vi "enumAttr.vi"() -> ()   [LabVIEW 2016]
uses:
  <vilib>/userdefined/High Color/IMAQdx.ctl
  <vilib>/vision/driver/IMAQdx.llb/IMAQdx Attribute Type.ctl
  <vilib>/vision/driver/NI_Vision_Acquisition_Software.lvlib
panel:
  in  "stop":bool
  out "error out":errorcluster
  out "Attribute Information Array":T2(array[cluster])
  in  "Session In":T3
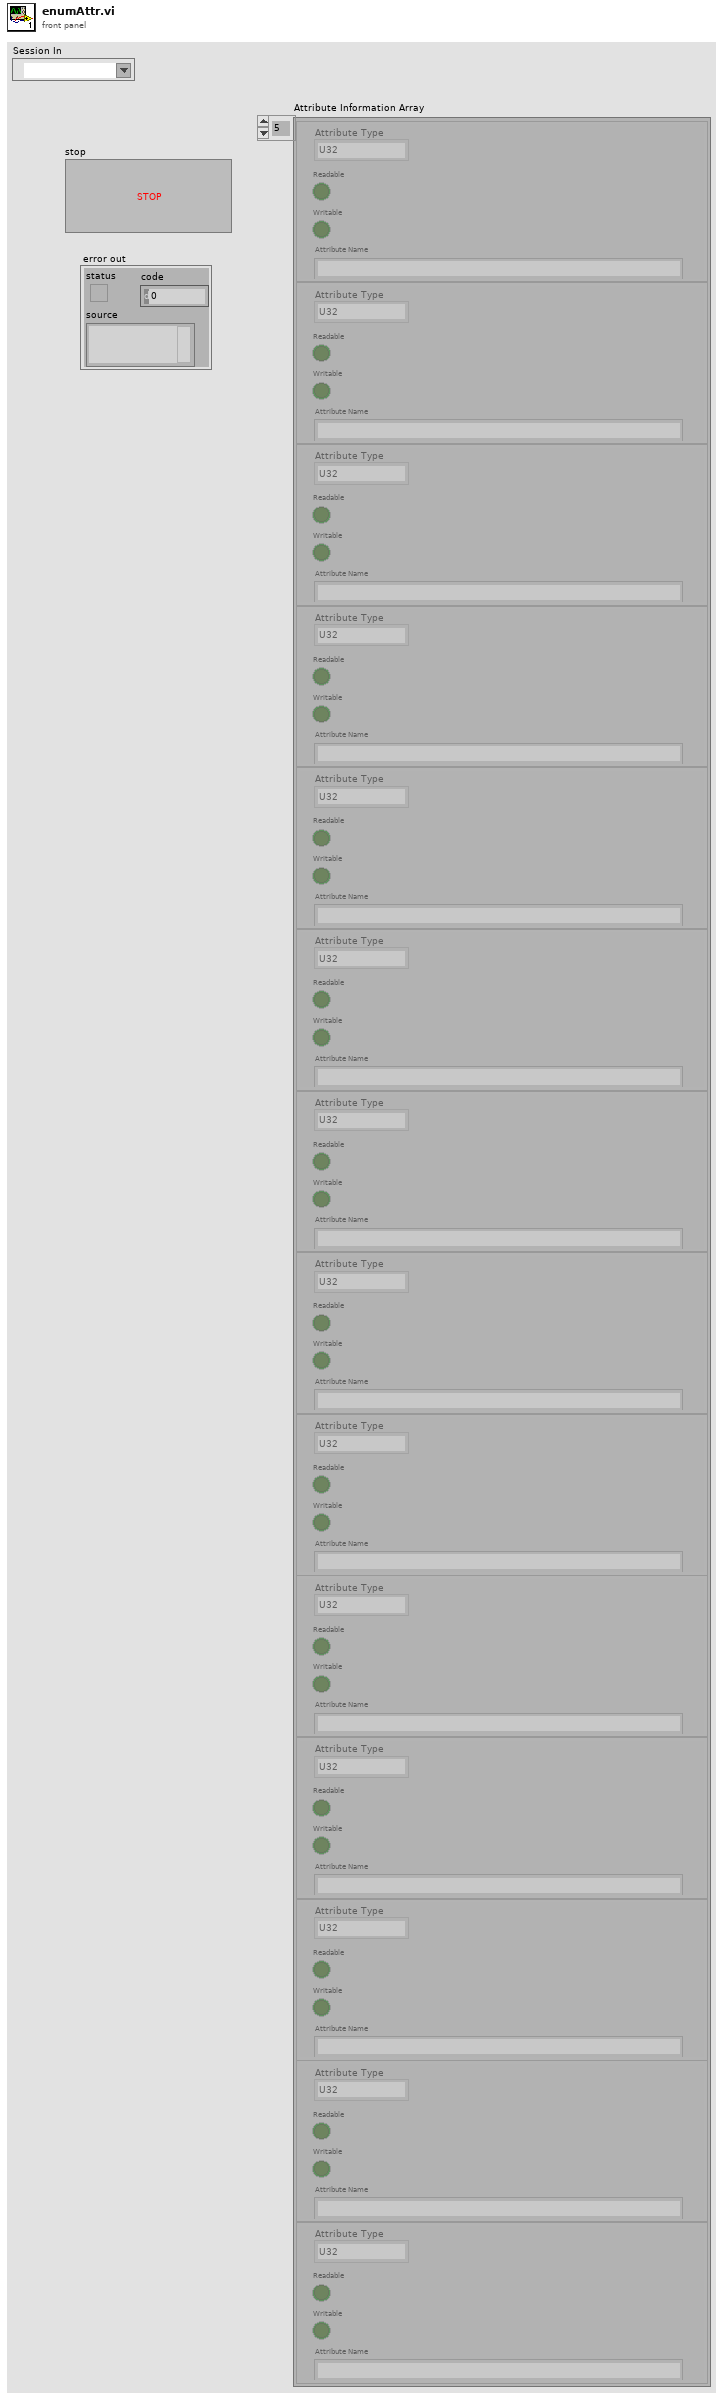
[diagram p1: front panel]
types:
  T1 = typedef "NI_Vision_Acquisition_Software.lvlib/IMAQdx Attribute Type.ctl" = enum32{"U32", "I64", "DBL", "String", "Enum", "Bool", "Command"}
  T2 = cluster{"Attribute Type":T1, "Readable":bool, "Writable":bool, "Attribute Name":string}[]
  T3 = typedef "IMAQdx.ctl" = refnum<k21>
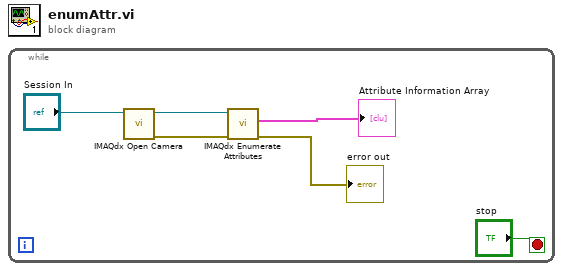
[diagram p0: block diagram]
diagram:
  n1 = while {
    stop <- "stop" stop-if-true
    n2 = call <vilib>:"IMAQdx Open Camera.vi"("Session In"="Session In") -> ("error out"=w4:errorcluster, "Session Out"=w5:T3)  [unwired: 9 in]
    n3 = call <vilib>:"IMAQdx Enumerate Attributes.vi"("error in"=w4, "Session In"=w5) -> ("error out"=→"error out":errorcluster, "Attribute Information Array"=→"Attribute Information Array":T2)  [unwired: 7 in, 1 out]
  }
